vi "MR.vi"() -> ()   [LabVIEW 2017]
panel:
  in  "OK Button":bool
  in  "Max Temp [°C]":u8(knob) scale=30.0..110.0
  out "Celsius Display":string
  out "Warning":bool
  out "Celsius":dbl(slide) scale=-50.0..110.0
  in  "Fahrenheit":dbl(slide) scale=-50.0..230.0
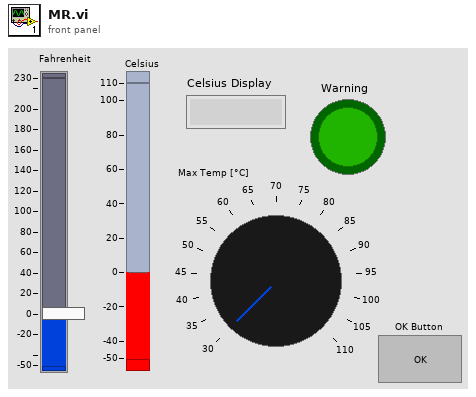
[diagram p1: front panel]
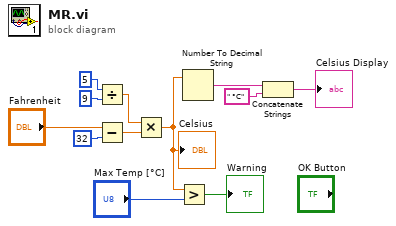
[diagram p0: block diagram]
diagram:
  n1 = Divide(x=5, y=9) -> (x/y=w8:dbl)
  n2 = Subtract(x="Fahrenheit", y=32) -> (x-y=w11:dbl)
  n3 = Multiply(x=w8, y=w11) -> (x*y=w2:dbl)
  "Celsius" <- w2
  n4 = Greater?(x=w2, y="Max Temp [°C]") -> (0:→"Warning":bool)
  n5 = Number To Decimal String(number=w2) -> (decimal integer string=w3:string)  [unwired: 1 in]
  n6 = Concatenate Strings(w3, " °C") -> (→"Celsius Display":string)
